vi "StackingSensorGet.vi"() -> (4 "Pos5":bool, 6 "Pos4":bool, 8 "Pos3":bool, 10 "Pos2":bool, 14 "Distance":dbl, 15 "Pos1":bool)   [LabVIEW 2014]
uses:
  Global Variables/Refnum Names.vi
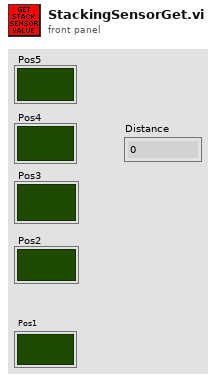
[diagram p1: front panel]
types:
  T1 = typedef "WPI_EncoderDevRef.ctl" = cluster{"DevStatus":errorcluster, "EncoderIndex":T2, "CounterIndex":T3, "DistancePerCount":dbl, "Decoding Type":T4}
  T2 = typedef "FPGA_EncoderIdx.ctl" = enum8{"Enc 0", "Enc 1", "Enc 2", "Enc 3", "Enc 4", "Enc 5", "Enc 6", "Enc 7", "Invalid"}
  T3 = typedef "FPGA_CounterCtrSystemIndex.ctl" = enum8{"Ctr 0", "Ctr 1", "Ctr 2", "Ctr 3", "Ctr 4", "Ctr 5", "Ctr 6", "Ctr 7", "Invalid"}
  T4 = typedef "WPI_EncoderType.ctl" = enum16{"1x", "2x", "4x"}
  T5 = typedef "WPI_DigitalInputDevRef.ctl" = cluster{"DevStatus":errorcluster, "DIO Channel":T6, "Controller":T7}
  T6 = typedef "FPGA_DIOChannel.ctl" = enum8{"DIO 0", "DIO 1", "DIO 2", "DIO 3", "DIO 4", "DIO 5", "DIO 6", "DIO 7", "DIO 8", "DIO 9", "DIO MXP 0", "DIO MXP 1", "DIO MXP 2", "DIO MXP 3", "DIO MXP 4", "DIO MXP 5", "DIO MXP 6", "DIO MXP 7", "DIO MXP 8", "DIO MXP 9", "DIO MXP 10", "DIO MXP 11", "DIO MXP 12", "DIO MXP 13", "DIO MXP 14", "DIO MXP 15", "Invalid"}
  T7 = typedef "FPGA_TypedefDigitalModule.ctl" = enum16{"Controller 1"}
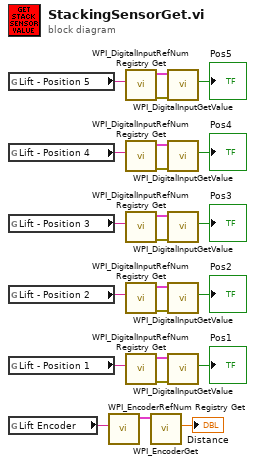
[diagram p0: block diagram]
diagram:
  n1 = global read "Refnum Names.vi" "Lift - Position 5"() -> (w14:string)
  n2 = global read "Refnum Names.vi" "Lift - Position 4"() -> (w15:string)
  n3 = global read "Refnum Names.vi" "Lift - Position 3"() -> (w16:string)
  n4 = global read "Refnum Names.vi" "Lift - Position 2"() -> (w17:string)
  n5 = global read "Refnum Names.vi" "Lift - Position 1"() -> (w18:string)
  n6 = global read "Refnum Names.vi" "Lift Encoder"() -> (w3:string)
  n7 = call <vilib>:"WPI_EncoderRefNum Registry Get.vi"("refnum name"=w3) -> ("EncoderDevRef"=w2:T1)  [unwired: 9 in, 1 out]
  n8 = call <vilib>:"WPI_DigitalInputRefNum Registry Get.vi"("refnum name"=w14) -> ("error out"=w4:errorcluster, "DigitalInputDevRef"=w5:T5)  [unwired: 9 in]
  n9 = call <vilib>:"WPI_DigitalInputRefNum Registry Get.vi"("refnum name"=w15) -> ("error out"=w9:errorcluster, "DigitalInputDevRef"=w10:T5)  [unwired: 9 in]
  n10 = call <vilib>:"WPI_DigitalInputRefNum Registry Get.vi"("refnum name"=w16) -> ("error out"=w6:errorcluster, "DigitalInputDevRef"=w11:T5)  [unwired: 9 in]
  n11 = call <vilib>:"WPI_DigitalInputRefNum Registry Get.vi"("refnum name"=w17) -> ("error out"=w7:errorcluster, "DigitalInputDevRef"=w12:T5)  [unwired: 9 in]
  n12 = call <vilib>:"WPI_DigitalInputRefNum Registry Get.vi"("refnum name"=w18) -> ("error out"=w8:errorcluster, "DigitalInputDevRef"=w13:T5)  [unwired: 9 in]
  n13 = call <vilib>:"WPI_EncoderGet.vi"("EncoderDevRef"=w2) -> ("Distance"=→"Distance":dbl)  [unwired: 5 in, 5 out]
  n14 = call <vilib>:"WPI_DigitalInputGetValue.vi"("error in (no error)"=w4, "DigitalInputDevRef"=w5) -> ("Value"=→"Pos5":bool)  [unwired: 7 in, 2 out]
  n15 = call <vilib>:"WPI_DigitalInputGetValue.vi"("error in (no error)"=w9, "DigitalInputDevRef"=w10) -> ("Value"=→"Pos4":bool)  [unwired: 7 in, 2 out]
  n16 = call <vilib>:"WPI_DigitalInputGetValue.vi"("error in (no error)"=w6, "DigitalInputDevRef"=w11) -> ("Value"=→"Pos3":bool)  [unwired: 7 in, 2 out]
  n17 = call <vilib>:"WPI_DigitalInputGetValue.vi"("error in (no error)"=w7, "DigitalInputDevRef"=w12) -> ("Value"=→"Pos2":bool)  [unwired: 7 in, 2 out]
  n18 = call <vilib>:"WPI_DigitalInputGetValue.vi"("error in (no error)"=w8, "DigitalInputDevRef"=w13) -> ("Value"=→"Pos1":bool)  [unwired: 7 in, 2 out]
